vi "read.vi"(8 "error in (no error)":errorcluster, 11 "MOXAIP in":refnum<class "MOXAIP.lvclass">) -> (0 "error out":errorcluster, 2 "Bytes":u8[](array[numeric]), 3 "MOXAIP out":refnum<class "MOXAIP.lvclass">)   [LabVIEW 2015, in "Serializer.lvlib" / "MOXAIP.lvclass"]
uses:
  MOXAIP.lvclass
  MOXAIP.lvclass/MOXAIP.ctl
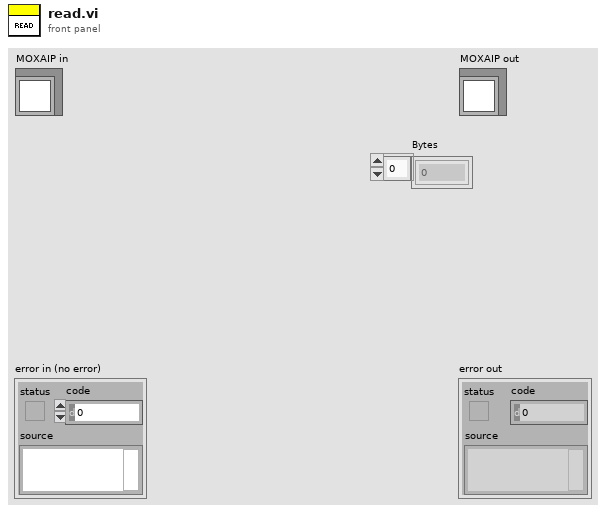
[diagram p1: front panel]
types:
  T1 = enum16{"Standard", "Buffered", "CRLF", "Immediate"}
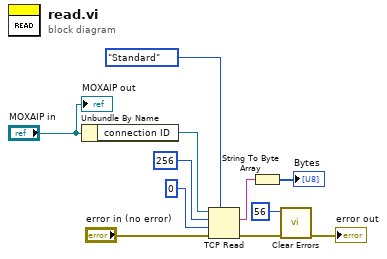
[diagram p0: block diagram]
diagram:
  n1 = Unbundle By Name("MOXAIP in") -> ("connection ID"=w11:refnum<k5>)
  n2 = TCP Read(connection ID=w11, bytes to read=256, error in (no error)="error in (no error)", 7:T1."Standard" ("mode (standard)"), 9:0 ("timeout ms (25000)")) -> (data out=w9:string, error out=w4:errorcluster)  [unwired: 1 out]
  n3 = String To Byte Array(string=w9) -> (unsigned byte array=→"Bytes":u8[])
  n4 = call <vilib>:"Clear Errors.vi"("error in (no error)"=w4, "specific error code to clear (0: all)"=56) -> ("error out"=→"error out":errorcluster)  [unwired: 4 in, 1 out]
  "MOXAIP out" <- "MOXAIP in"
